vi "LDF Get Signal Value.vi"(7 "pValue":dbl, 9 "pSignalName":string, 10 "pFrameName":string, 11 "LDFHandle":u64) -> (1 "pSignalName out":string, 2 "pFrameName out":string, 3 "function return":i32, 5 "pValue out":dbl)   [LabVIEW 2010, in "ldf_parser.lvlib"]
doc: "int WINAPI LDF_GetSignalValue(long long LDFHandle, char* pFrameName, char* pSignalName, double *pValue);"
uses:
  ldf_parser.lvlib
  USB2XXX/trunk/USB2XXX/USB2XXX/vs2019/Release/USB2XXX.dll
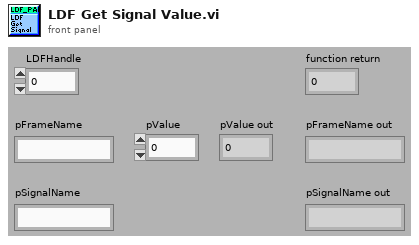
[diagram p1: front panel]
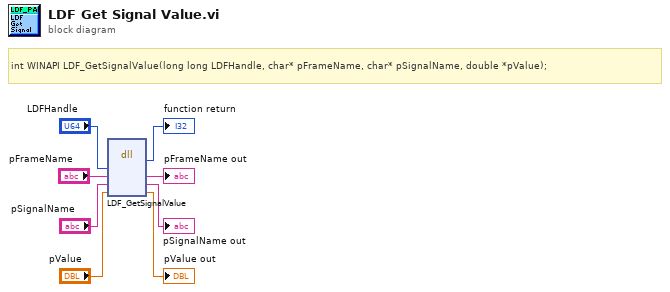
[diagram p0: block diagram]
diagram:
  # "int WINAPI LDF_GetSignalValue(long long LDFHandle, char* pFrameName, char* pSignalName, double *pValue);"
  n1 = dll-call lib="E:/Projects/USB2XXX/trunk/USB2XXX/USB2XXX/vs2019/Release/USB2XXX.*" fn="LDF_GetSignalValue"("LDFHandle"="LDFHandle", "pFrameName"="pFrameName", "pSignalName"="pSignalName", "pValue"="pValue") -> (→"function return":i32, "pFrameName"=→"pFrameName out":string, "pSignalName"=→"pSignalName out":string, "pValue"=→"pValue out":dbl)  [unwired: 4 in, 2 out]
